vi "photons_counter.vi"(9 "timetags":u32[](array[numeric]), 10 "start_read":u32[](array[numeric]), 11 "stop_read":u32[](array[numeric])) -> (3 "photons_counts":i32[](array[numeric]))   [LabVIEW 2018]
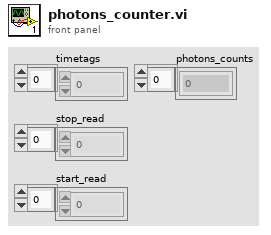
[diagram p1: front panel]
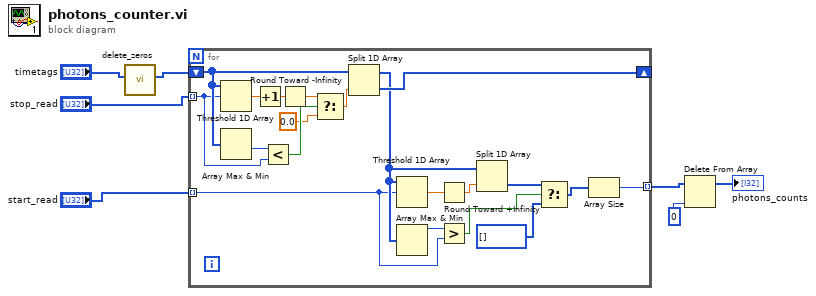
[diagram p0: block diagram]
diagram:
  n1 = call "delete_zeros.vi"("array_in"="timetags") -> ("array_out"=w2:u32[])  [unwired: 10 in]
  n2 = for {
    tunnel: "start_read" -> [w19] mode=indexing
    tunnel: "stop_read" -> [w13] mode=indexing
    shift-right: [w27] -> _
    shift-left: w2 -> [w15]
    tunnel: [w26] -> w6 mode=indexing
    n3 = Threshold 1D Array(2:w13, 3:w15) -> (0:w24:dbl)  [unwired: 1 in]
    n4 = Array Max & Min(array=w15) -> (min value=w14:u32)  [unwired: 3 out]
    n5 = Increment(x=w24) -> (x+1=w23:dbl)
    n6 = Less?(x=w14, y=w13) -> (x < y?=w10:bool)
    n7 = Round Toward -Infinity(1:w23) -> (0:w12:dbl)
    n8 = Select(t=w12, s=w10, f=0.0 ("index")) -> (s? t:f=w11:dbl)
    n9 = Split 1D Array(array=w15, index=w11) -> (first subarray=w21:u32[], second subarray=w27:u32[])
    n10 = Threshold 1D Array(2:w19, 3:w21) -> (0:w22:dbl)  [unwired: 1 in]
    n11 = Array Max & Min(array=w21) -> (max value=w20:u32)  [unwired: 3 out]
    n12 = Round Toward +Infinity(x=w22) -> (ceil(x): smallest int >= x=w25:dbl)
    n13 = Greater?(x=w20, y=w19) -> (0:w18:bool)
    n14 = Split 1D Array(array=w21, index=w25) -> (second subarray=w17:u32[])  [unwired: 1 out]
    n15 = Select(t=w17, s=w18, f=u32[] [] ("second subarray")) -> (s? t:f=w8:u32[])
    n16 = Array Size(array=w8) -> (size(s)=w26:i32)
  }
  n17 = Delete From Array(array=w6, index=0) -> (array with subset deleted=→"photons_counts":i32[])  [unwired: 1 in, 1 out]
